vi "lab4-3.vi"() -> ()   [LabVIEW 2018]
uses:
  <vilib>/DAQmx/create/channels.llb/DAQmx Create Channel (CO-Pulse Generation-Frequency).vi
panel:
  in  "Frequency":dbl
  out "error out":errorcluster
  in  "stop":bool
  in  "error in":errorcluster
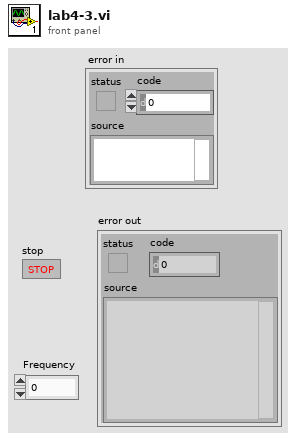
[diagram p1: front panel]
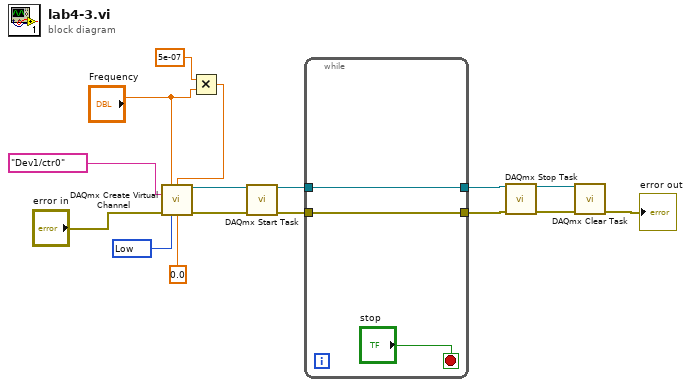
[diagram p0: block diagram]
diagram:
  w15 = 10214 items=["High"=10192, "Low"=10214] ("idle state")
  n1 = Multiply(x=5e-07, y="Frequency") -> (x*y=w13:dbl)
  n2 = call-poly <vilib>:"DAQmx Create Virtual Channel.vi"("frequency"="Frequency", "duty cycle"=w13, "counter"=tag "Dev1/ctr0", "error in"="error in", "idle state"=w15, "initial delay"=0.0) -> ("task out"=w2:refnum<k21>, "error out"=w1:errorcluster)  [unwired: 8 in]
  n3 = call <vilib>:"DAQmx Start Task.vi"("task/channels in"=w2, "error in"=w1) -> ("task out"=w10:refnum<k21>, "error out"=w8:errorcluster)  [unwired: 12 in]
  n4 = while {
    tunnel: [w18] -> w11
    tunnel: w10 -> [w18]
    tunnel: [w17] -> w9
    tunnel: w8 -> [w17]
    stop <- "stop" stop-if-true
  }
  n5 = call <vilib>:"DAQmx Stop Task.vi"("task/channels in"=w11, "error in"=w9) -> ("task out"=w7:refnum<k21>, "error out"=w6:errorcluster)  [unwired: 12 in]
  n6 = call <vilib>:"DAQmx Clear Task.vi"("task in"=w7, "error in"=w6) -> ("error out"=→"error out":errorcluster)  [unwired: 13 in]
